vi "MPP.OnOff.vi"(8 "error in (no error)":errorcluster, 10 "ON?":bool, 11 "VISA Refnum in":refnum<visa-resource-name>) -> (0 "error out":errorcluster, 3 "VISA Refnum out":refnum<visa-resource-name>)   [LabVIEW 2020, in "main.lvlib"]
uses:
  main.lvlib
  <instrlib>/HH PLA Series/HH PLA Series.lvlib
panel:
  out "state":string
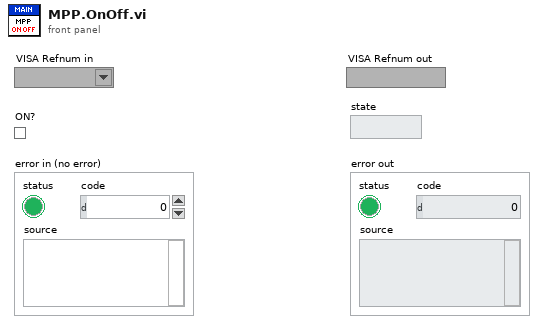
[diagram p1: front panel]
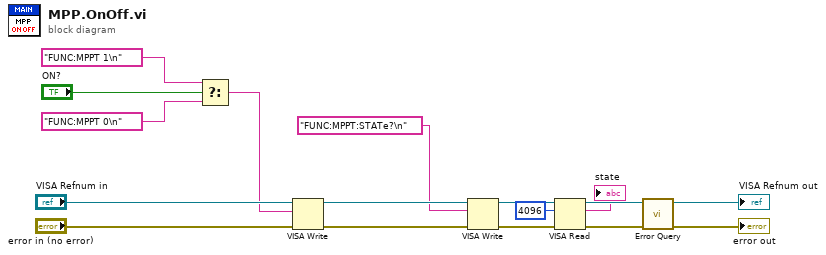
[diagram p0: block diagram]
diagram:
  n1 = Select(t="FUNC:MPPT 1\n" ("write buffer"), s="ON?", f="FUNC:MPPT 0\n" ("write buffer")) -> (s? t:f=w9:string)
  n2 = VISA Write(VISA resource name="VISA Refnum in", write buffer=w9, error in (no error)="error in (no error)") -> (VISA resource name out=w7:refnum<visa-resource-name>, error out=w15:errorcluster)  [unwired: 1 out]
  n3 = VISA Write(VISA resource name=w7, write buffer="FUNC:MPPT:STATe?\n", error in (no error)=w15) -> (VISA resource name out=w4:refnum<visa-resource-name>, error out=w8:errorcluster)  [unwired: 1 out]
  n4 = VISA Read(VISA resource name=w4, byte count=u32 4096, error in (no error)=w8) -> (VISA resource name out=w3:refnum<visa-resource-name>, read buffer=→"state":string, error out=w5:errorcluster)  [unwired: 1 out]
  n5 = call <instrlib>:"Error Query.vi"("error in (no error)"=w5, "VISA resource name"=w3) -> ("error out"=→"error out":errorcluster, "VISA resource name out"=→"VISA Refnum out":refnum<visa-resource-name>)  [unwired: 6 in, 2 out]
